vi "AbortTest.vi"(8 "error in (no error)":errorcluster, 11 "reference in":refnum<class "Test_Base.lvclass">) -> (0 "error out":errorcluster, 3 "reference in":refnum<class "Test_Base.lvclass">)   [LabVIEW 2022 SP3, in "Test_Base.lvlib" / "Test_Base.lvclass"]
uses:
  Test_Base.lvclass
  Components/TestView_Base.lvlibp/ViewStatus.ctl
  Components/TestView_Base.lvlibp/TestView_Base.lvclass
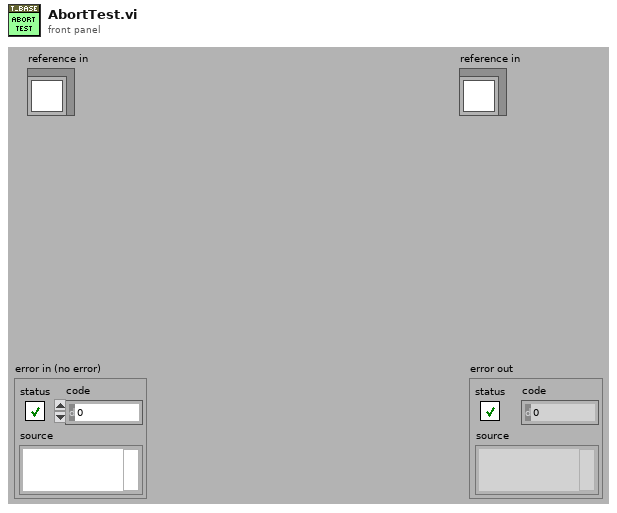
[diagram p1: front panel]
types:
  T1 = typedef "TestView_Base.lvlibp/TestView_Base.lvclass/ViewStatus.ctl" = enum16{"Testing", "Ready", "Logout", "Login", "PASS", "FAIL", "FAULT", "ABORTED"}
  T2 = typedef "Test_Base.lvlib/Test_Base.lvclass/ObjectAttributes.ctl" = cluster{"Config":T3, "UUTIndex":i32, "Serial":string, "Batch":string, "MES":refnum<class "MES_Base.lvclass">, "TestView":refnum<class "TestView_Base.lvclass">, "LoggedIn":bool, "Abort":bool}
  T3 = typedef "Test_Base.lvlib/Test_Base.lvclass/Config.ctl" = cluster{"ContinueOnFail":bool}
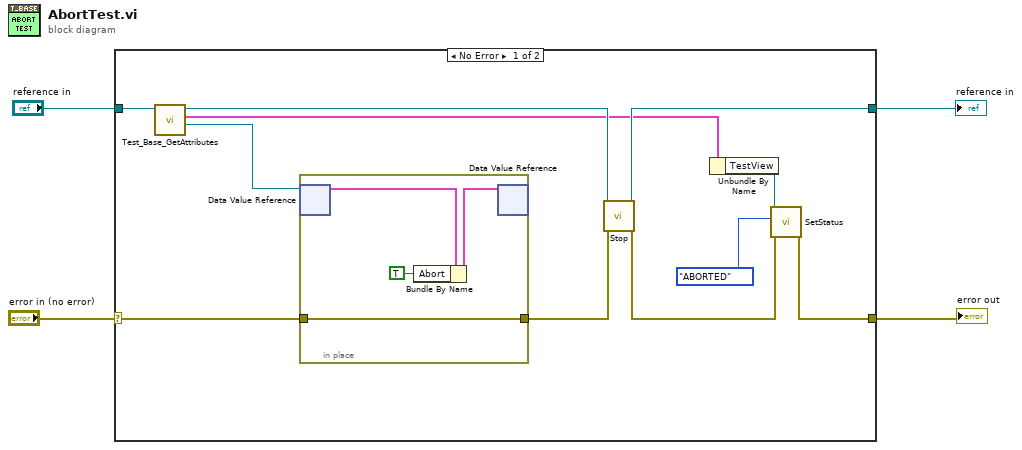
[diagram p0: block diagram]
diagram:
  n1 = case shown="No Error" "error in (no error)" {
    selector: "error in (no error)" -> [w10 w21]
    tunnel: [w7 w21] -> w3
    tunnel: [w12 w20] -> w1
    tunnel: "reference in" -> [w15 w20]
    frame No Error {
      n2 = call "Test_Base_GetAttributes.vi"("reference in"=w15) -> ("DataRef"=w14:refnum<data-value>, "Data"=w6:T2, "reference out"=w13:refnum<class "Test_Base.lvclass">)  [unwired: 7 in, 1 out]
      n3 = in-place {
        in-place-border: [w16] -> w11
        in-place-border: w10 -> [w16]
        n4 = in-place-dvr #1(w14) -> (w19:T2)  [unwired: 1 out]
        n5 = Bundle By Name(cluster=w19, "Abort"=TRUE) -> (w18:T2)
        n6 = in-place-dvr #1(w18) -> ()  [unwired: 2 out]
      }
      n7 = call-dynamic "Stop.vi"("error in (no error)"=w11, "reference in"=w13) -> ("error out"=w8:errorcluster, "reference in"=w12:refnum<class "Test_Base.lvclass">)  [unwired: 8 in]
      n8 = Unbundle By Name(w6) -> ("TestView"=w5:refnum<class "TestView_Base.lvclass">)
      n9 = call-dynamic "SetStatus.vi"("error in (no error)"=w8, "Status"=ViewStatus."ABORTED", "reference in"=w5) -> ("error out"=w7:errorcluster)  [unwired: 7 in, 1 out]
    }
    frame Error {
    }
  }
  "error out" <- w3
  "reference in" <- w1
